vi "Convert IP Address.vi"(8 "error in (no error)":errorcluster, 11 "IP":string) -> (0 "error out":errorcluster, 3 "net address":u32 format="%.0x")   [LabVIEW 2021, in "Networking_CIF_U.lvlib"]
uses:
  Networking_CIF_U.lvlib
  Typedef/Errors.ctl
  SubVIs/Network Error Core.vi
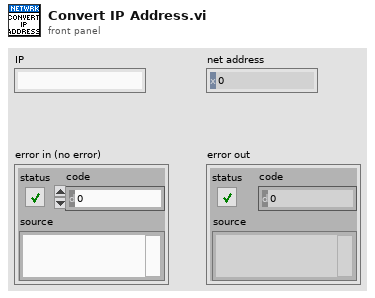
[diagram p1: front panel]
types:
  T1 = typedef "Networking_CIF_U.lvlib/Errors.ctl" = enum16{"Invalid IP Address", "No Subnet Match Found", "Error Finding Port", "No Ping Response", "Nettools Needed", "Error Checking Port"}
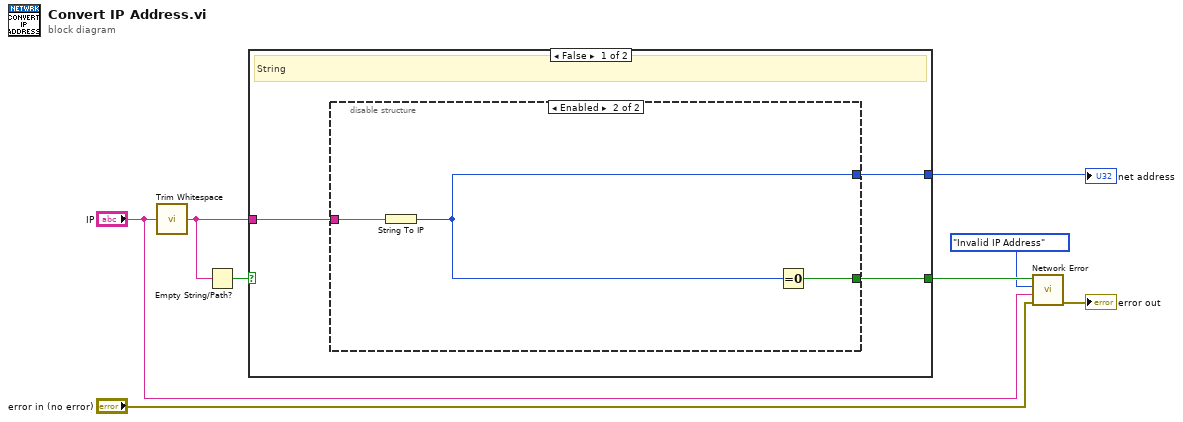
[diagram p0: block diagram]
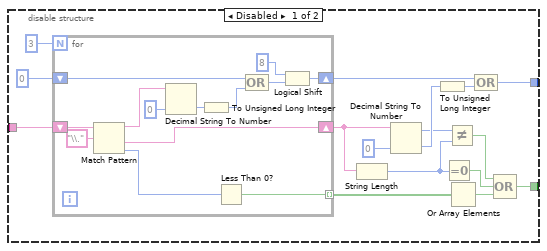
[diagram p2: hidden frame]
diagram:
  n1 = call <vilib>:"Trim Whitespace.vi"("string"="IP") -> ("trimmed string"=w2:string)  [unwired: 1 in]
  n2 = Empty String/Path?(string/path=w2) -> (empty?=w1:bool)
  n3 = case shown="False" w1 {
    selector: w1 -> [_ w44]
    tunnel: [w11 _] -> w8
    tunnel: [w10 w44] -> w7
    tunnel: w2 -> [w9 _]
    frame False {
      # "String"
      n4 = disable-structure shown="Enabled" {
        disable-tunnel: [w18 w42] -> w11
        disable-tunnel: [w17 w41] -> w10
        disable-tunnel: w9 -> [w12 w43]
        frame Disabled {
          n5 = for {
            N: 3 -> [_]
            shift-right: [w36] -> w25
            shift-left: w12 -> [w40]
            tunnel: [w34] -> w23 mode=indexing
            shift-right: [w29] -> w20
            shift-left: u32 0 -> [w33]
            n6 = Match Pattern(string=w40, regular expression="\\.") -> (before substring=w38:string, after substring=w36:string, offset past match=w35:i32)  [unwired: 1 in, 1 out]
            n7 = Decimal String To Number(string=w38, default (0L)=u8 0 ("default (0 I32)")) -> (number=w32:u8)  [unwired: 1 in, 1 out]
            n8 = To Unsigned Long Integer(number=w32) -> (unsigned 32bit integer=w28:u32)
            n9 = Less Than 0?(x=w35) -> (x < 0?=w34:bool)
            n10 = Compound Arithmetic op=OR(w33, w28) -> (w31:u32)
            n11 = Logical Shift(y=i16 8, x=w31) -> (x << y=w29:u32)
          }
          n12 = String Length(string=w25) -> (length=w15:i32)
          n13 = Decimal String To Number(string=w25, default (0L)=u8 0 ("default (0 I32)")) -> (offset past number=w16:i32, number=w19:u8)  [unwired: 1 in]
          n14 = To Unsigned Long Integer(number=w19) -> (unsigned 32bit integer=w13:u32)
          n15 = Equal To 0?(x=w15) -> (x = 0?=w24:bool)
          n16 = Not Equal?(x=w16, y=w15) -> (x != y?=w14:bool)
          n17 = Or Array Elements(Boolean array=w23) -> (logical OR=w22:bool)
          n18 = Compound Arithmetic op=OR(w20, w13) -> (w18:u32)
          n19 = Compound Arithmetic op=OR(w14, w24, w22) -> (w17:bool)
        }
        frame Enabled {
          n20 = String To IP(1:w43) -> (0:w42:u32)
          n21 = Equal To 0?(x=w42) -> (x = 0?=w41:bool)
        }
      }
    }
    frame True {
      # "Empty IP.  Prefer to error on empty since this is normally an error (default will return a local IP address)"
    }
  }
  "net address" <- w8
  n22 = call "Network Error.vi"("error in (no error)"="error in (no error)", "String to Append"="IP", "Error"=Errors."Invalid IP Address", "Insert Error"=w7) -> ("error out"=→"error out":errorcluster)  [unwired: 7 in]
